vi "Close Workspace Control Refs.vi"(11 "State Variables in":T1={"UI.Refs"={"Chart"=refnum, "Manual Value"=refnum, "Manual Output"=refnum, "Revert"=refnum, "Apply"=refnum, "Setpoint"=refnum, "Autoscale X"=refnum, "Autoscale Y"=refnum, "Hold"=refnum, "Manual Control"=refnum, "Device"=refnum}, "Addon.GUID"="", "Addon.Name"="", "Addon.Type"=enum."Industrial", "Data.UDPEngineQueue"=refnum, "Data.Found?"=FALSE, "Data.UDPChannels"=[], "Data.PreviousValues"=[], "Data.SlowChannels"=[], "Data.PendingChange?"=FALSE, "CachedData.UserEvent"=refnum, "CachedData.Data"={"Path"=""}, "Addon.Connected?"=FALSE, "NIVS.SysDefRoot"=refnum, "NIVS.Workspace"=refnum, "NIVS.UserEventRefs"={"Event Registration Refnum"=refnum, "SystemChangeEventRef"=refnum}, "NIVS.SystemStateRefs"={"CustDatRef"=refnum, "EvtRef"=refnum, "Target State User Event"=refnum}, "NIVS.LaunchRef"=refnum, "Setpoint Range"={"Min"=0.0, "Max"=0.0}, "Output Range"={"Min"=0.0, "Max"=0.0}}) -> ()   [LabVIEW 2019, in "Control Workspace Object.lvlib"]
uses:
  Control Workspace Object.lvlib
  Types/Workspace Object State Variables.ctl
  Types/UI.Refs.ctl
  Types/UDP Streaming Command Cluster.ctl
  Types/UDP Streaming State.ctl
  <vilib>/NI VeriStand/Display Template Support/DisplayTemplateSupport.llb/enum_Display Template Handler Minimal To Workspace.ctl
  Types/Workspace Object Cached Settings.ctl
  NationalInstruments.VeriStand.SystemStorage
  <vilib>/NI VeriStand/Execution/Workspace/WorkspaceAPI.ctl
  NationalInstruments.VeriStand.ClientAPI
  <vilib>/NI VeriStand/Display Template Support/DisplayTemplateSupport.llb/enum_Display Template Handler Minimal To Widget Msg.ctl
  <vilib>/NI VeriStand/Execution/Workspace/SystemStateRegEventRef.ctl
  <vilib>/NI VeriStand/Execution/Workspace/Target State Info.ctl
  <vilib>/NI VeriStand/Execution/Workspace/Target State.ctl
  <vilib>/NI VeriStand/Execution/Workspace/SystemStateEventRef.ctl
  <vilib>/NI VeriStand/Execution/Workspace/NI_VS Workspace ExecutionAPI.lvlib
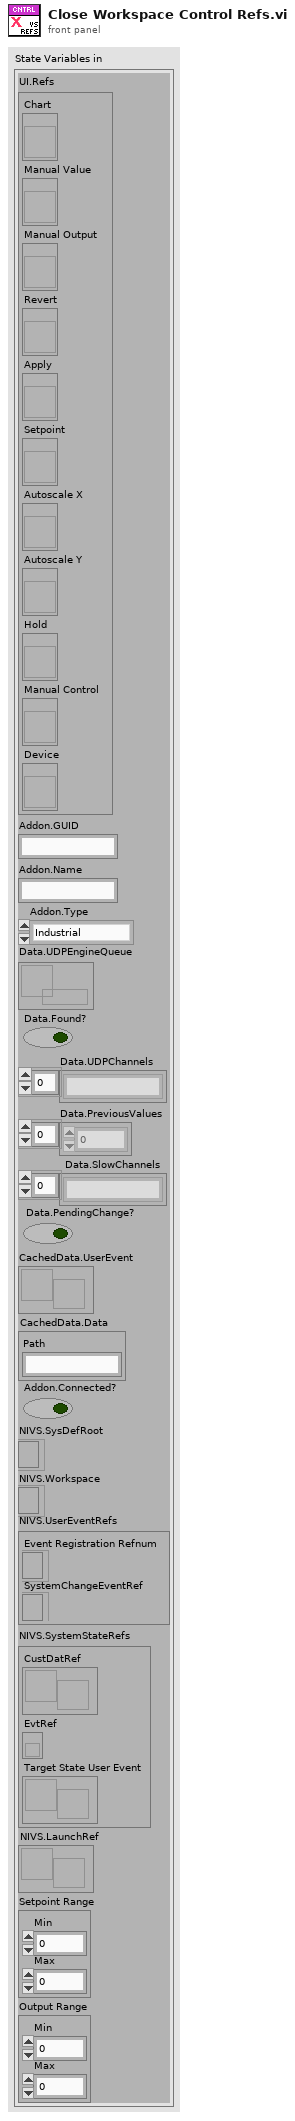
[diagram p1: front panel]
types:
  T1 = typedef "Control Workspace Object.lvlib/Workspace Object State Variables.ctl" = cluster{"UI.Refs":T2, "Addon.GUID":string, "Addon.Name":string, "Addon.Type":enum16{"PID", "Industrial"}, "Data.UDPEngineQueue":refnum<queue>, "Data.Found?":bool, "Data.UDPChannels":string[], "Data.PreviousValues":dbl[], "Data.SlowChannels":string[], "Data.PendingChange?":bool, "CachedData.UserEvent":refnum<user-event>, "CachedData.Data":T3, "Addon.Connected?":bool, "NIVS.SysDefRoot":refnum<k24>, "NIVS.Workspace":T4, "NIVS.UserEventRefs":cluster{"Event Registration Refnum":refnum<event-registration>, "SystemChangeEventRef":T5}, "NIVS.SystemStateRefs":T6, "NIVS.LaunchRef":refnum<user-event>, "Setpoint Range":cluster{"Min":dbl, "Max":dbl}, "Output Range":cluster{"Min":dbl, "Max":dbl}}
  T2 = typedef "Control Workspace Object.lvlib/UI.Refs.ctl" = cluster{"Chart":refnum<vi>, "Manual Value":refnum<vi>, "Manual Output":refnum<vi>, "Revert":refnum<vi>, "Apply":refnum<vi>, "Setpoint":refnum<vi>, "Autoscale X":refnum<vi>, "Autoscale Y":refnum<vi>, "Hold":refnum<vi>, "Manual Control":refnum<vi>, "Device":refnum<vi>}
  T3 = typedef "Control Workspace Object.lvlib/Workspace Object Cached Settings.ctl" = cluster{"Path":string}
  T4 = typedef "NI_VS Workspace ExecutionAPI.lvlib/WorkspaceAPI.ctl" = refnum<k24>
  T5 = typedef "NI_VS Workspace ExecutionAPI.lvlib/SystemStateRegEventRef.ctl" = refnum<event-registration>
  T6 = typedef "NI_VS Workspace ExecutionAPI.lvlib/SystemStateEventRef.ctl" = cluster{"CustDatRef":refnum<user-event>, "EvtRef":refnum<k27>, "Target State User Event":refnum<user-event>}
  T7 = cluster{"Event Registration Refnum":refnum<event-registration>, "SystemChangeEventRef":T5}
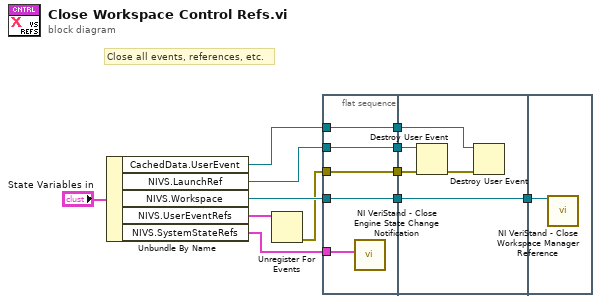
[diagram p0: block diagram]
diagram:
  # "Close all events, references, etc."
  n1 = Unbundle By Name("State Variables in") -> ("CachedData.UserEvent"=w7:refnum<user-event>, "NIVS.LaunchRef"=w6:refnum<user-event>, "NIVS.Workspace"=w4:T4, "NIVS.UserEventRefs"=w3:T7, "NIVS.SystemStateRefs"=w5:T6)
  n2 = Unregister For Events(event registration refnum=w3) -> (error out=w1:errorcluster)  [unwired: 1 in]
  n3 = flat-sequence {
    tunnel: w4 -> [w14]
    tunnel: w5 -> [w13]
    tunnel: w7 -> [w15]
    tunnel: w6 -> [w16]
    tunnel: w1 -> [w17]
    tunnel: [w17] -> w12
    tunnel: [w16] -> w11
    tunnel: [w15] -> w10
    tunnel: [w14] -> w9
    tunnel: w12 -> [w21]
    tunnel: w11 -> [w22]
    tunnel: w10 -> [w19]
    tunnel: w9 -> [w18]
    tunnel: [w18] -> w8
    tunnel: w8 -> [w23]
    frame #0 {
      n4 = call <vilib>:"NI VeriStand - Close Engine State Change Notification.vi"("SystemStateRefs"=w13) -> ()  [unwired: 10 in, 1 out]
    }
    frame #1 {
      n5 = Destroy User Event(user event=w22, error in=w21) -> (error out=w20:errorcluster)
      n6 = Destroy User Event(user event=w19, error in=w20) -> ()  [unwired: 1 out]
    }
    frame #2 {
      n7 = call <vilib>:"NI VeriStand - Close Workspace Manager Reference.vi"("WorkspaceManager"=w23) -> ()  [unwired: 10 in, 1 out]
    }
  }
